vi "Launcher.vi"() -> ()   [LabVIEW 2021, in "Echo Broadcast Test With Server Manager.lvlib"]
uses:
  Echo Broadcast Test With Server Manager.lvlib
  WS Test Server Subscriber/WS Test Server Subscriber.lvclass
  C:/Program Files/National Instruments/LabVIEW 2021/vi.lib/ActorFramework/Actor/Actor.lvclass
  WebSocket Actor/WebSocket Server Manager/WebSocket Server Manager.lvclass
  WS Test Server Subscriber/WS Test Server Subscriber.lvclass/WS Test Server Subscriber.ctl
  <vilib>/ActorFramework/Message Enqueuer/Message Enqueuer.lvclass/Message Enqueuer.ctl
  WS Test Client Subscriber/WS Test Client Subscriber.lvclass
  WS Test Server Subscriber/properties/Write WebSocket Server Manager Enqueuer.vi
  <vilib>/ActorFramework/Message Enqueuer/Enqueue.vi
  <vilib>/ActorFramework/Stop Msg/Stop Msg.lvclass
  C:/Program Files/National Instruments/LabVIEW 2021/vi.lib/ActorFramework/Message/Message.lvclass
  <vilib>/ActorFramework/Message Priority Queue/Priority Enqueue.vi
  <vilib>/ActorFramework/Actor/Actor.lvclass
  C:/Program Files/National Instruments/LabVIEW 2021/vi.lib/MGI/Monitored Actor/Monitored Actor/Monitored Actor/Monitored Actor.lvclass
  C:/Projects/Shared Libraries/WebSocket Actor/Tests/Echo Broadcast Test With Server Manager/WS Test Client Subscriber/WS Test Client Subscriber.lvclass
panel:
  in  "Stop Server":bool
  in  "Number of Clients":i32=3
  out "error out":errorcluster
  # "In this example we will use the Server Manager Actor Infrastructure to launch a WebSocket server and we will illustrate a bidirectional communication between the WebSocket server and clients. \nWe launch one server that will define the /echo/ service. Then a user selectable number of clients can be launched. From such clients messages to the servers can be sent on the specified service. The server will echo back the message to the client. The server can broadcast messages to the clients. One can choose to send a series of messages at a certain time frequency. \nInstructions to execute the example;\n1. Run this VI\n2. Wait that the Server and Client GUI appear\n3. use the GUIs to exchange messages\n4. Exit the Client GUI form their GUI themselves\n5. Stop the servers from this VI"
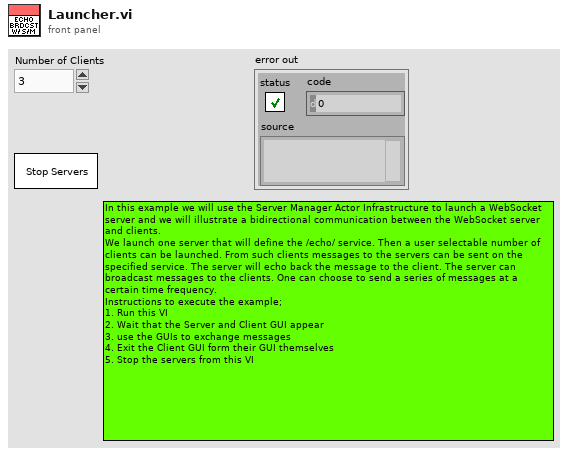
[diagram p1: front panel]
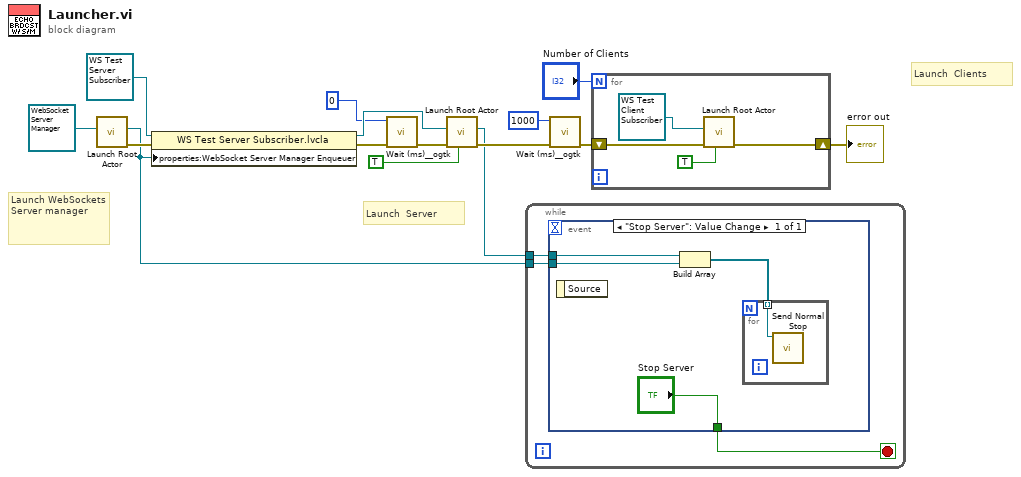
[diagram p0: block diagram]
diagram:
  # "Launch  Clients"
  # "Launch  Server"
  # "Launch WebSockets Server manager"
  n1 = call <vilib>:"Launch Root Actor.vi"("Actor"=refnum<class "WebSocket Server Manager.lvclass"> refnum ("WebSocket Actors.lvlib:WebSocket Server Manager.lvclass")) -> ("error out"=w9:errorcluster, "Actor's Enqueuer"=w5:refnum<class "Message Enqueuer.lvclass">)  [unwired: 9 in]
  n2 = property class="WS Test Server Subscriber.lvcla"(reference=refnum<class "WS Test Server Subscriber.lvclass"> refnum ("WS Full LabVIEW Test.lvlib:WS Test Server.lvclass"), error in=w9, "properties:WebSocket Server Manager Enqueuer"=w5) -> (reference out=w10:refnum<class "WS Test Server Subscriber.lvclass">, error out=w3:errorcluster)
  n3 = call <userlib>:"Wait (ms)__ogtk.vi"("error in (no error)"=w3, "milliseconds to wait"=u32 0) -> ("error out"=w2:errorcluster)  [unwired: 8 in, 1 out]
  n4 = call <vilib>:"Launch Root Actor.vi"("Open Actor Core front panel? (F)"=TRUE, "error in (no error)"=w2, "Actor"=w10) -> ("error out"=w13:errorcluster, "Actor's Enqueuer"=w4:refnum<class "Message Enqueuer.lvclass">)  [unwired: 7 in]
  n5 = while {
    tunnel: w5 -> [w18]
    tunnel: w4 -> [w16]
    stop <- w17 stop-if-true
    n6 = event shown="[0] \"Stop Server\": Value Change" {
      selector: _ -> [_]
      dyn-events: _ -> [_]
      timeout: _ -> [_]
      tunnel: w18 -> [w22]
      tunnel: ["Stop Server"] -> w17
      tunnel: w16 -> [w19]
      event "Stop Server": Value Change {
        n7 = event-data() -> ()  [unwired: 1 in, 1 out]
        n8 = Build Array(w19, w22) -> (w20:refnum<class "Message Enqueuer.lvclass">[])
        n9 = for {
          tunnel: w20 -> [w23] mode=indexing
          n10 = call <vilib>:"Send Normal Stop.vi"("Message Enqueuer"=w23) -> ()  [unwired: 10 in, 1 out]
        }
      }
    }
  }
  n11 = call <userlib>:"Wait (ms)__ogtk.vi"("error in (no error)"=w13, "milliseconds to wait"=u32 1000) -> ("error out"=w8:errorcluster)  [unwired: 8 in, 1 out]
  n12 = for {
    N: "Number of Clients" -> [_]
    shift-right: [w24] -> w12
    shift-left: w8 -> [w25]
    n13 = call <vilib>:"Launch Root Actor.vi"("Open Actor Core front panel? (F)"=TRUE, "error in (no error)"=w25, "Actor"=refnum<class "WS Test Client Subscriber.lvclass"> refnum ("WS Full LabVIEW Test.lvlib:WS Test Client.lvclass")) -> ("error out"=w24:errorcluster)  [unwired: 7 in, 1 out]
  }
  "error out" <- w12
